vi "i2clib_writeread.vi"(6 "recv_size":i32, 8 "error in (no error)":errorcluster, 9 "send_data":u8[](array[numeric]), 10 "dev_addr":u8, 11 "I2C Reference":i32) -> (0 "error out":errorcluster, 2 "recv_data":u8[](array[numeric]), 3 "I2C Reference Out":i32)   [LabVIEW 2017]
uses:
  <vilib>/Utility/error.llb/Error Cluster From Error Code.vi
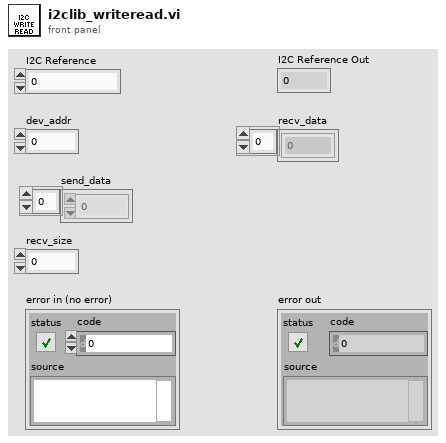
[diagram p1: front panel]
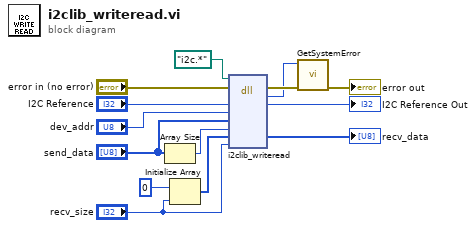
[diagram p0: block diagram]
diagram:
  n1 = Array Size(array="send_data") -> (size(s)=w4:i32)
  n2 = Initialize Array(i8 0 ("dev_addr"), "recv_size") -> (w8:i8[])
  n3 = dll-call lib="?" fn="i2clib_writeread"(path in=path "i2c.*", error in="error in (no error)", "handle"="I2C Reference", "dev_addr"="dev_addr", "send_buf"="send_data", "send_size"=w4, "recv_buf"=w8, "revc_size"="recv_size") -> (error out=w3:errorcluster, "return type"=w2:i32, "handle"=→"I2C Reference Out":i32, "recv_buf"=→"recv_data":i8[])  [unwired: 5 in, 1 out]
  n4 = call <vilib>:"GetSystemError.vi"("error in (no error)"=w3, "Retval"=w2) -> ("error out"=→"error out":errorcluster)  [unwired: 9 in]
